vi "CMD_DEC.vi"(6 "Gantry in":refnum<class "Gantry.lvclass">, 8 "error in (no error)":errorcluster, 10 "Arguments":string[](array[string]), 11 "gScript Interpreter in":refnum<class "gScript Interpreter.lvclass">) -> (0 "error out":errorcluster, 3 "gScript Interpreter out":refnum<class "gScript Interpreter.lvclass">, 4 "Gantry out":refnum<class "Gantry.lvclass">)   [LabVIEW 2022 SP3, in "gScript Interpreter.lvclass"]
uses:
  gScript Interpreter.lvclass
  gScript Interpreter.lvclass/gScript Interpreter.ctl
  Type Definitions/Memory Cell Type Enum.ctl
  Type Definitions/Memory Cell.ctl
  Shared Components/Gantry Class/Gantry.lvclass
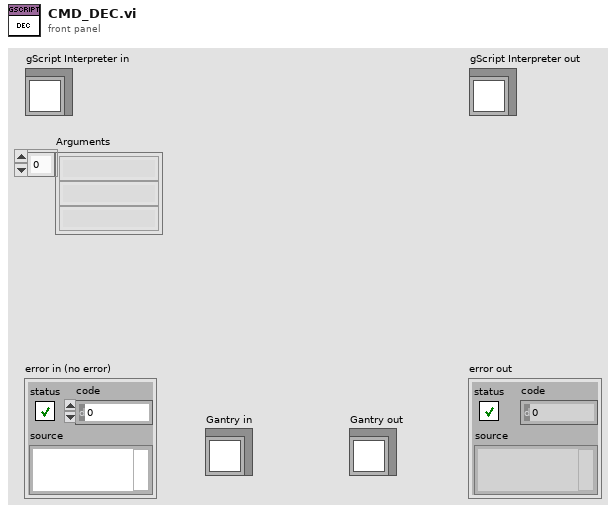
[diagram p1: front panel]
types:
  T1 = typedef "Memory Cell.ctl" = cluster{"type":T2, "x":dbl, "y":dbl, "z":dbl, "w":dbl}
  T2 = typedef "Memory Cell Type Enum.ctl" = enum16{"integer", "float", "vector", "rotation"}
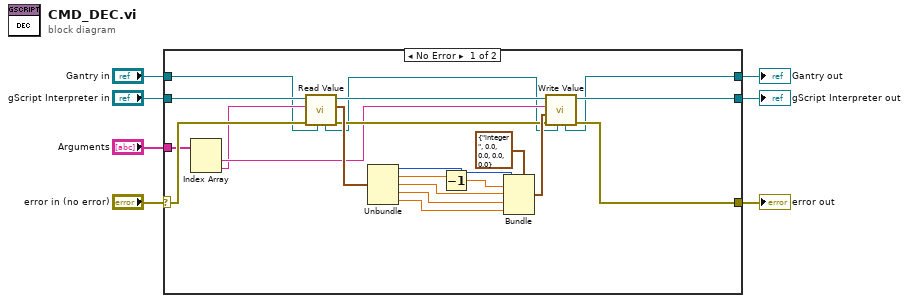
[diagram p0: block diagram]
diagram:
  n1 = case shown="No Error" "error in (no error)" {
    selector: "error in (no error)" -> [w19 w31]
    tunnel: [w22 w31] -> w4
    tunnel: [w23 w30] -> w3
    tunnel: "gScript Interpreter in" -> [w20 w30]
    tunnel: "Arguments" -> [w13 _]
    tunnel: "Gantry in" -> [w10 w29]
    tunnel: [w8 w29] -> w1
    frame No Error {
      n2 = Index Array(array=w13) -> (element #1=w12:string, element #2=w11:string)  [unwired: 2 in]
      n3 = call-dynamic "Read Value.vi"("Gantry in"=w10, "error in (no error)"=w19, "String in"=w11, "gScript Interpreter in"=w20) -> ("error out"=w24:errorcluster, "Memory Cell"=w28:T1, "gScript Interpreter out"=w27:refnum<class "gScript Interpreter.lvclass">, "Gantry out"=w9:refnum<class "Gantry.lvclass">)  [unwired: 4 in]
      n4 = Unbundle(w28) -> ("type"=w21:T2, "x"=w18:dbl, "y"=w16:dbl, "z"=w15:dbl, "w"=w14:dbl)
      n5 = Decrement(x=w18) -> (x-1=w17:dbl)
      n6 = Bundle(cluster=T1 {"type"=enum."integer", "x"=0.0, "y"=0.0, "z"=0.0, "w"=0.0} ("Memory Cell"), "type"=w21, "x"=w17, "y"=w16, "z"=w15, "w"=w14) -> (w25:T1)
      n7 = call-dynamic "Write Value.vi"("Gantry in"=w9, "error in (no error)"=w24, "Value"=w25, "Address"=w12, "gScript Interpreter in"=w27) -> ("error out"=w22:errorcluster, "gScript Interpreter out"=w23:refnum<class "gScript Interpreter.lvclass">, "Gantry out"=w8:refnum<class "Gantry.lvclass">)  [unwired: 4 in]
    }
    frame Error {
    }
  }
  "error out" <- w4
  "gScript Interpreter out" <- w3
  "Gantry out" <- w1
